vi "Create.vi"(5 "Agent Fixture in":refnum<class "Agent Fixture.lvclass">, 8 "error in (no error)":errorcluster) -> (0 "error out":errorcluster, 3 "Agent Fixture":refnum<class "Agent Fixture.lvclass">)   [LabVIEW 2013, in "libssh2_integration_tests.lvlib" / "Agent Fixture.lvclass"]
uses:
  Agent Fixture.lvclass
  Agent Fixture.lvclass/Agent Fixture.ctl
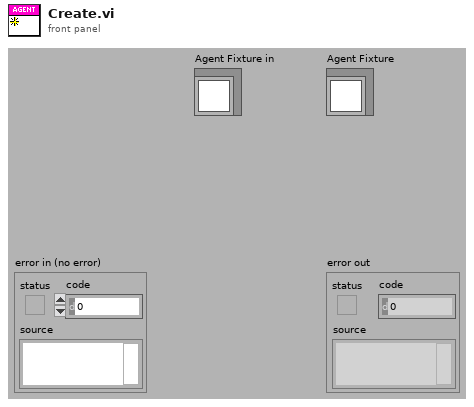
[diagram p1: front panel]
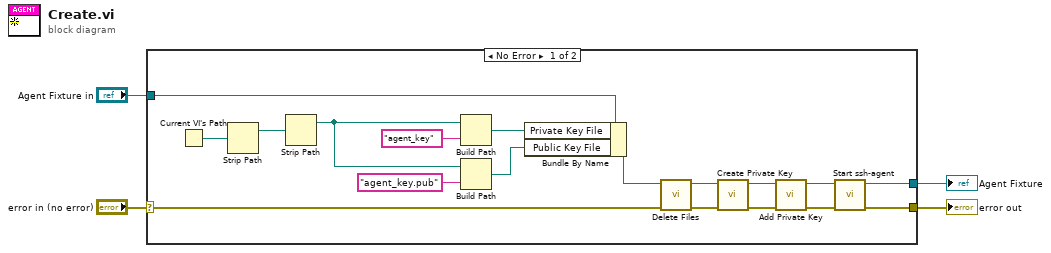
[diagram p0: block diagram]
diagram:
  n1 = case shown="No Error" "error in (no error)" {
    selector: "error in (no error)" -> [w13 w24]
    tunnel: [w22 w24] -> w3
    tunnel: [w20 w23] -> w1
    tunnel: "Agent Fixture in" -> [w21 w23]
    frame No Error {
      n2 = Current VI's Path() -> (path=w18:path)
      n3 = Strip Path(path=w18) -> (stripped path=w17:path)  [unwired: 1 out]
      n4 = Strip Path(path=w17) -> (stripped path=w6:path)  [unwired: 1 out]
      n5 = Build Path(base path=w6, name or relative path="agent_key") -> (appended path=w16:path)
      n6 = Build Path(base path=w6, name or relative path="agent_key.pub") -> (appended path=w5:path)
      n7 = Bundle By Name(cluster=w21, "Private Key File"=w16, "Public Key File"=w5) -> (w15:refnum<class "Agent Fixture.lvclass">)
      n8 = call "Delete Files.vi"("error in (no error)"=w13, "Agent Fixture in"=w15) -> ("error out"=w14:errorcluster, "Agent Fixture out"=w11:refnum<class "Agent Fixture.lvclass">)  [unwired: 8 in]
      n9 = call "Create Private Key.vi"("error in (no error)"=w14, "Agent Fixture in"=w11) -> ("error out"=w12:errorcluster, "Agent Fixture out"=w9:refnum<class "Agent Fixture.lvclass">)  [unwired: 8 in]
      n10 = call "Add Private Key.vi"("error in (no error)"=w12, "Agent Fixture in"=w9) -> ("error out"=w10:errorcluster, "Agent Fixture out"=w8:refnum<class "Agent Fixture.lvclass">)  [unwired: 8 in]
      n11 = call "Start ssh-agent.vi"("error in (no error)"=w10, "Agent Fixture in"=w8) -> ("error out"=w22:errorcluster, "Agent Fixture out"=w20:refnum<class "Agent Fixture.lvclass">)  [unwired: 8 in]
    }
    frame Error {
    }
  }
  "error out" <- w3
  "Agent Fixture" <- w1
